vi "PH_Numbers.Conflict Checker.vi"(1 "Input 2":i32, 2 "Input 1":i32) -> (0 "Result":i32)   [LabVIEW 2014, in "PH_Common.lvlib"]
doc: "This VI calculates the logical output of two incoming informations in the following sense:\n\nAt \"Input 1\" (In 1) and \"Input 2\" (In 2) the 0, 1 and 2 are expected; at \"Result\" you will get 0, 1, 2, 3:\n\nIn 1 and/or In 2 = 0 -> Result = 0\nIn 1 = 2 and In 2 = 1 -> Result = 1\nIn 1 = 1 and In 2 = 2 -> Result = 2\nIn 1 = In 2 -> Result = 3\nelse -> Result = 0"
uses:
  PH_Common.lvlib
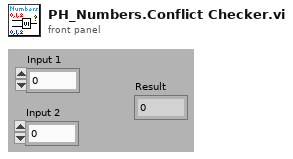
[diagram p1: front panel]
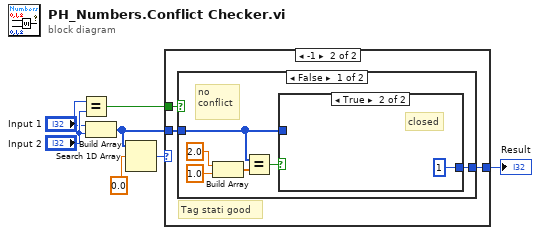
[diagram p0: block diagram]
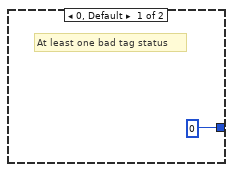
[diagram p2: hidden frame]
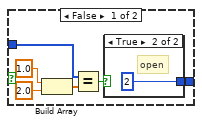
[diagram p3: hidden frame]
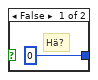
[diagram p4: hidden frame]
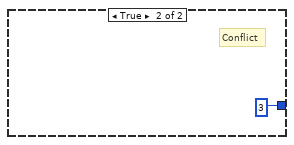
[diagram p5: hidden frame]
diagram:
  n1 = Equal?(x="Input 1", y="Input 2") -> (x = y?=w5:bool)
  n2 = Build Array("Input 1", "Input 2") -> (w4:i32[])
  n3 = Search 1D Array(1D array=w4, element=0.0) -> (index of element=w2:i32)  [unwired: 1 in]
  n4 = case shown="-1" w2 {
    tunnel: w4 -> [_ w10]
    tunnel: w5 -> [_ w11]
    tunnel: [0 w9] -> w3
    frame 0, Default {
      # "At least one bad tag status"
    }
    frame -1 {
      # "Tag stati good"
      n5 = case shown="False" w11 {
        tunnel: w10 -> [w13 _]
        tunnel: [w12 3] -> w9
        frame False {
          # "no\nconflict"
          n6 = Build Array(2.0 ("element"), 1.0 ("element")) -> (w14:dbl[])
          n7 = Equal?(x=w13, y=w14) -> (x = y?=w15:bool)
          n8 = case shown="True" w15 {
            tunnel: w13 -> [w19 _]
            tunnel: [w18 1] -> w12
            frame False {
              n9 = Build Array(1.0 ("element"), 2.0 ("element")) -> (w21:dbl[])
              n10 = Equal?(x=w19, y=w21) -> (x = y?=w20:bool)
              n11 = case shown="True" w20 {
                tunnel: [0 2] -> w18
                frame False {
                  # "Hä?"
                }
                frame True {
                  # "open"
                }
              }
            }
            frame True {
              # "closed"
            }
          }
        }
        frame True {
          # "Conflict"
        }
      }
    }
  }
  "Result" <- w3
